vi "LoggerDaemon.vi"(6 "Write delay (ms)":u32=1000, 8 "error in (no error)":errorcluster, 9 "Stop Cmd Reference":refnum<data-value>, 10 "Log Message Queue":refnum<queue>, 11 "File path":path) -> (0 "error out":errorcluster)   [LabVIEW 2011, in "Logger.lvclass"]
doc: "Daemon (running in the background) which consistently checks the internal queue for new data to log. When there is some, it writes to the text file."
uses:
  Logger.lvclass
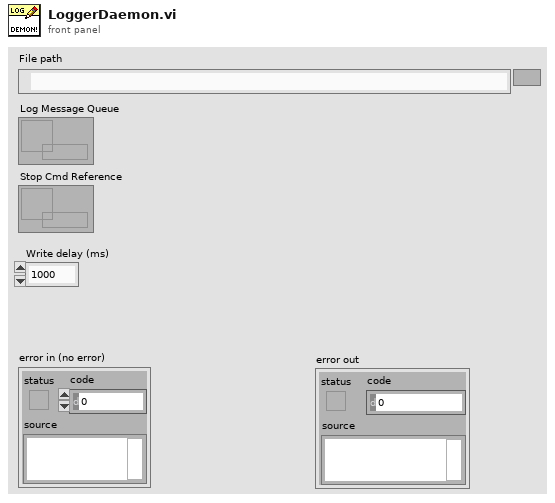
[diagram p1: front panel]
types:
  T1 = enum16{"open", "replace", "create", "open or create", "replace or create", "replace or create with confirmation"}
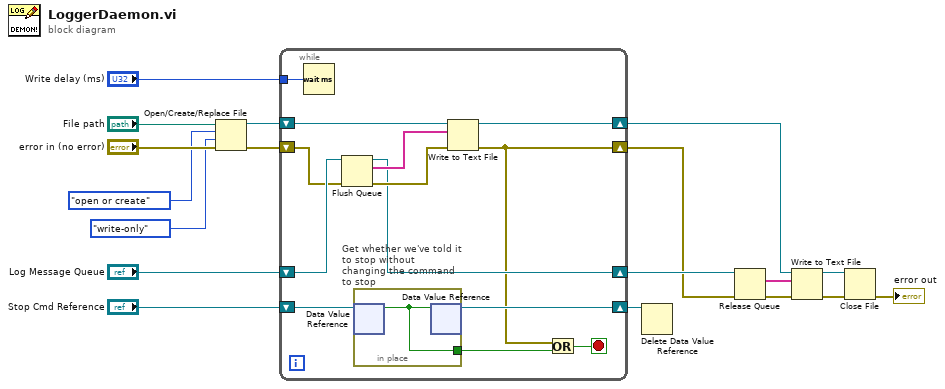
[diagram p0: block diagram]
diagram:
  n1 = Open/Create/Replace File(file path (use dialog)="File path", error in="error in (no error)", operation (0:open)=T1."open or create", access (0:read/write)=enum16{"read/write", "read-only", "write-only"}."write-only") -> (refnum out=w9:refnum<file>, error out=w8:errorcluster)  [unwired: 2 in, 1 out]
  n2 = while {
    shift-right: [w30] -> w17
    shift-left: "Stop Cmd Reference" -> [w31]
    tunnel: "Write delay (ms)" -> [w29]
    shift-right: [w22] -> w14
    shift-left: "Log Message Queue" -> [w28]
    shift-right: [w23] -> w5
    shift-left: w9 -> [w26]
    shift-right: [w19] -> w1
    shift-left: w8 -> [w27]
    stop <- w20 stop-if-true
    n3 = Wait (ms)(milliseconds to wait=w29) -> ()  [unwired: 1 out]
    n4 = Flush Queue(queue=w28, error in (no error)=w27) -> (queue out=w22:refnum<queue>, remaining elements=w25:string[], error out=w24:errorcluster)
    n5 = in-place "Get whether we've told it to stop without\nchanging the command to stop" {
      in-place-border: [w32] -> w21
      n6 = in-place-dvr #1(w31) -> (w32:bool)  [unwired: 1 out]
      n7 = in-place-dvr #1(w32) -> (w30:refnum<data-value>)  [unwired: 1 out]
    }
    n8 = Write to Text File(file (use dialog)=w26, text=w25, error in=w24) -> (refnum out=w23:refnum<file>, error out=w19:errorcluster)  [unwired: 1 in, 1 out]
    n9 = Or(x=w19, y=w21) -> (x .or. y?=w20:bool)
  }
  n10 = Delete Data Value Reference(data value reference=w17) -> ()  [unwired: 1 in, 2 out]
  n11 = Release Queue(queue=w14, error in (no error)=w1) -> (remaining elements=w6:string[], error out=w7:errorcluster)  [unwired: 1 in, 1 out]
  n12 = Write to Text File(file (use dialog)=w5, text=w6, error in=w7) -> (refnum out=w4:refnum<file>, error out=w3:errorcluster)  [unwired: 1 in, 1 out]
  n13 = Close File(refnum=w4, error in=w3) -> (error out=→"error out":errorcluster)  [unwired: 1 out]
